vi "AB_RW_Source_Encpwd.vi"(0 "input String":string) -> (2 "output String":string)   [LabVIEW 2020]
panel:
  in  "Line separator (\\n)":string="\n"
  # "Controls are hidden"
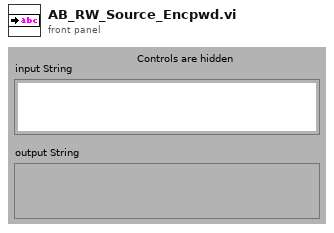
[diagram p1: front panel]
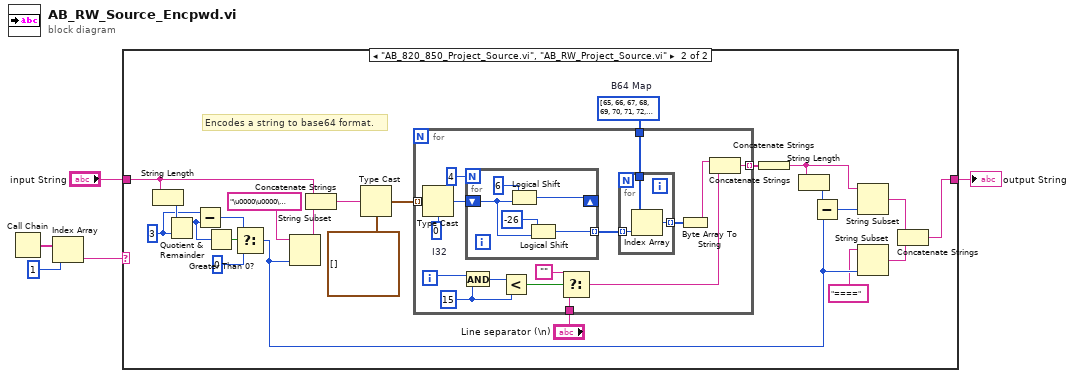
[diagram p0: block diagram]
diagram:
  n1 = Call Chain() -> (call chain=w3:string[])
  n2 = Index Array(array=w3, index=1) -> (element=w1:string)
  n3 = case shown="\"AB_820_850_Project_Source.vi\", \"AB_RW_Project_Source.vi\"" w1 {
    tunnel: "input String" -> [w6 w27]
    tunnel: [w6 w10] -> w4
    frame "False", Default {
    }
    frame "AB_820_850_Project_Source.vi", "AB_RW_Project_Source.vi" {
      w17 = u8[] [65, 66, 67, 68, 69, 70, 71, 72, 73, 74, 75, 76, 77, 78, 79, 80, 81, 82, 83, 84, 85, 86, 87, 88, 89, 90, 97, 98, 99, 100, 101, 102, 103, 104, 105, 106, 107, 108, 109, 110, 111, 112, 113, 114, 115, 116, 117, 118, 119, 120, 121, 122, 48, 49, 50, 51, 52, 53, 54, 55, 56, 57, 43, 47]  # B64 Map
      w23 = 3 ("y")
      # "Encodes a string to base64 format."
      n4 = String Length(string=w27) -> (length=w24:i32)
      n5 = Quotient & Remainder(x=w24, y=w23) -> (x-y*floor(x/y)=w22:i32)  [unwired: 1 out]
      n6 = Subtract(x=w23, y=w22) -> (x-y=w19:i32)
      n7 = Greater Than 0?(x=w22) -> (x > 0?=w21:bool)
      n8 = Select(t=w19, s=w21, f=0 ("y")) -> (s? t:f=w14:i32)
      n9 = String Subset(string="\u0000\u0000\u0000\u0000", length (rest)=w14) -> (substring=w28:string)  [unwired: 1 in]
      n10 = Concatenate Strings(w27, w28) -> (w26:string)
      n11 = Type Cast(type=cluster{"u8":u8, "u8":u8, "u8":u8}[] [], x=w26) -> (*(type *) &x=w18:cluster{"u8":u8, "u8":u8, "u8":u8}[])
      n12 = for {
        tunnel: w18 -> [w45] mode=indexing
        tunnel: w17 -> [w39]
        tunnel: "Line separator (\\n)" -> [w32]
        tunnel: [w30] -> w8 mode=indexing
        i -> [w35]
        w36 = 15 ("x")
        w44 = 0  # I32
        n13 = Type Cast(type=w44, x=w45) -> (*(type *) &x=w43:i32)
        n14 = And(x=w35, y=w36) -> (x .and. y?=w37:i32)
        n15 = for {
          N: 4 -> [_]
          shift-right: [w53] -> _
          shift-left: w43 -> [w50]
          tunnel: [w49] -> w40 mode=indexing
          n16 = Logical Shift(y=6, x=w50) -> (x << y=w53:i32)
          n17 = Logical Shift(y=-26, x=w50) -> (x << y=w49:i32)
        }
        n18 = Less?(x=w37, y=w36) -> (x < y?=w34:bool)
        n19 = Select(t="", s=w34, f=w32) -> (s? t:f=w31:string)
        n20 = for {
          tunnel: w40 -> [w48] mode=indexing
          tunnel: w39 -> [w47]
          tunnel: [w46] -> w38 mode=indexing
          n21 = Index Array(array=w47, index=w48) -> (element=w46:u8)
        }
        n22 = Byte Array To String(unsigned byte array=w38) -> (string=w42:string)
        n23 = Concatenate Strings(w42, w31) -> (w30:string)
      }
      n24 = Concatenate Strings(w8) -> (w7:string)
      n25 = String Length(string=w7) -> (length=w16:i32)
      n26 = Subtract(x=w16, y=w14) -> (x-y=w15:i32)
      n27 = String Subset(string=w7, length (rest)=w15) -> (substring=w12:string)  [unwired: 1 in]
      n28 = String Subset(string="====", length (rest)=w14) -> (substring=w11:string)  [unwired: 1 in]
      n29 = Concatenate Strings(w12, w11) -> (w10:string)
    }
  }
  "output String" <- w4
